vi "lvstyx_read_all_path_hex.vi"(7 "Log? (T)":bool=TRUE, 8 "error in (no error)":errorcluster, 10 "path":string, 11 "client ptr":u32) -> (0 "error out":errorcluster, 2 "uint32":u32, 3 "dup client ptr":u32)   [LabVIEW 2010, in "lib1299.lvlib"]
uses:
  lib1299.lvlib
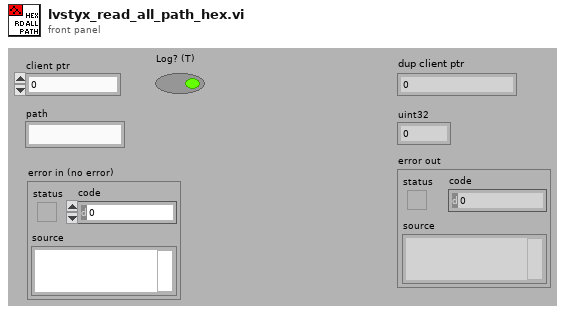
[diagram p1: front panel]
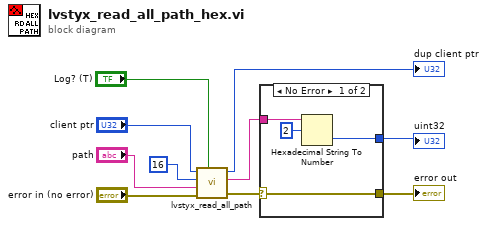
[diagram p0: block diagram]
diagram:
  n1 = call "lvstyx_read_all_path.vi"("Log? (T)"="Log? (T)", "error in (no error)"="error in (no error)", "path"="path", "lim"=16, "client ptr"="client ptr") -> ("error out"=w10:errorcluster, "buf"=w9:string, "dup client ptr"=→"dup client ptr":u32)  [unwired: 4 in]
  n2 = case shown="No Error" w10 {
    selector: w10 -> [w11 w15]
    tunnel: w9 -> [w14 _]
    tunnel: [w12 _] -> w8
    tunnel: [w11 w15] -> w5
    frame No Error {
      n3 = Hexadecimal String To Number(string=w14, offset=2) -> (number=w12:u32)  [unwired: 1 in, 1 out]
    }
    frame Error {
    }
  }
  "uint32" <- w8
  "error out" <- w5
